vi "Oscillo2graph2024.vi"() -> ()   [LabVIEW 2023]
panel:
  in  "Marker_Size":string
  out "Color Box 5":u32(colorbox)
  out "Color Box 4":u32(colorbox)
  out "Color Box 3":u32(colorbox)
  out "Color Box 2":u32(colorbox)
  out "Color Box":u32(colorbox)
  out "error out":errorcluster
  out "Corner color":u32(colorbox)
  out "Colors traces":string
  out "standard output":string
  out "CLUT":u32[](array[numeric])
  in  "Path":path
  in  "style of points":string
  out "PnG picture":picture
  out "Pixmap vraie couleurs":u32[](array[numeric])
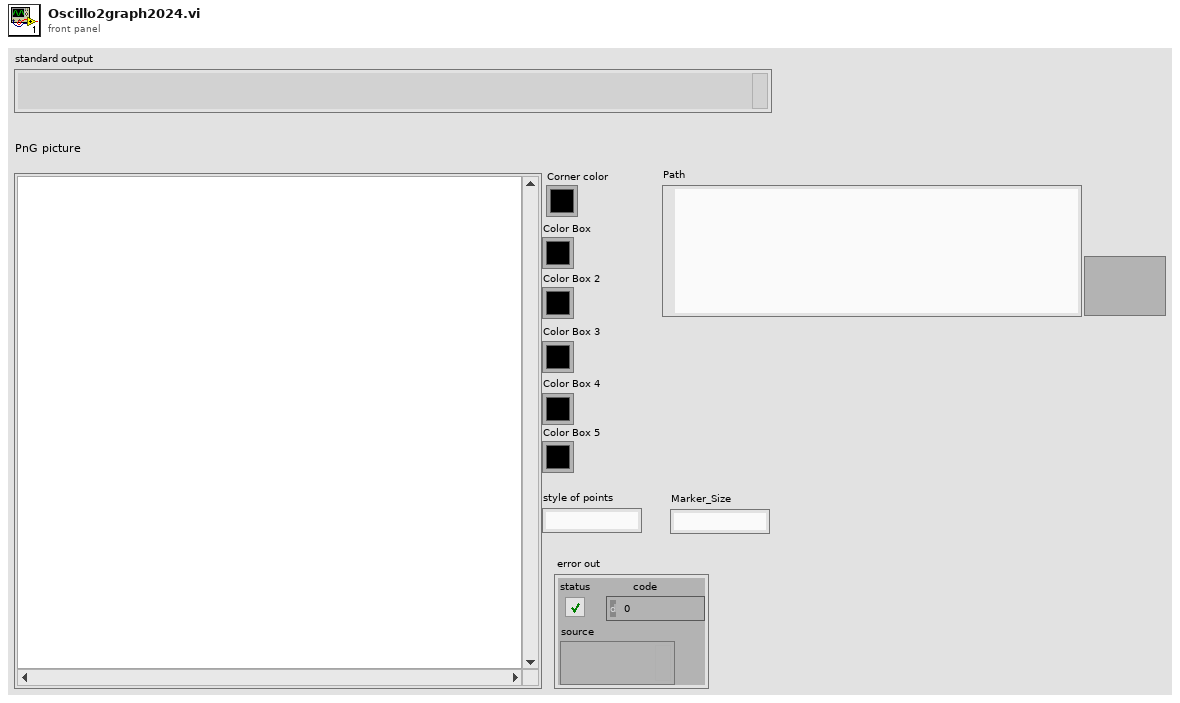
[diagram p1: front panel]
types:
  T1 = cluster{"[0]":u32, "[1]":u32, "[2]":u32, "[3]":u32, "[4]":u32, "[5]":u32, "[6]":u32, "[7]":u32, "[8]":u32}
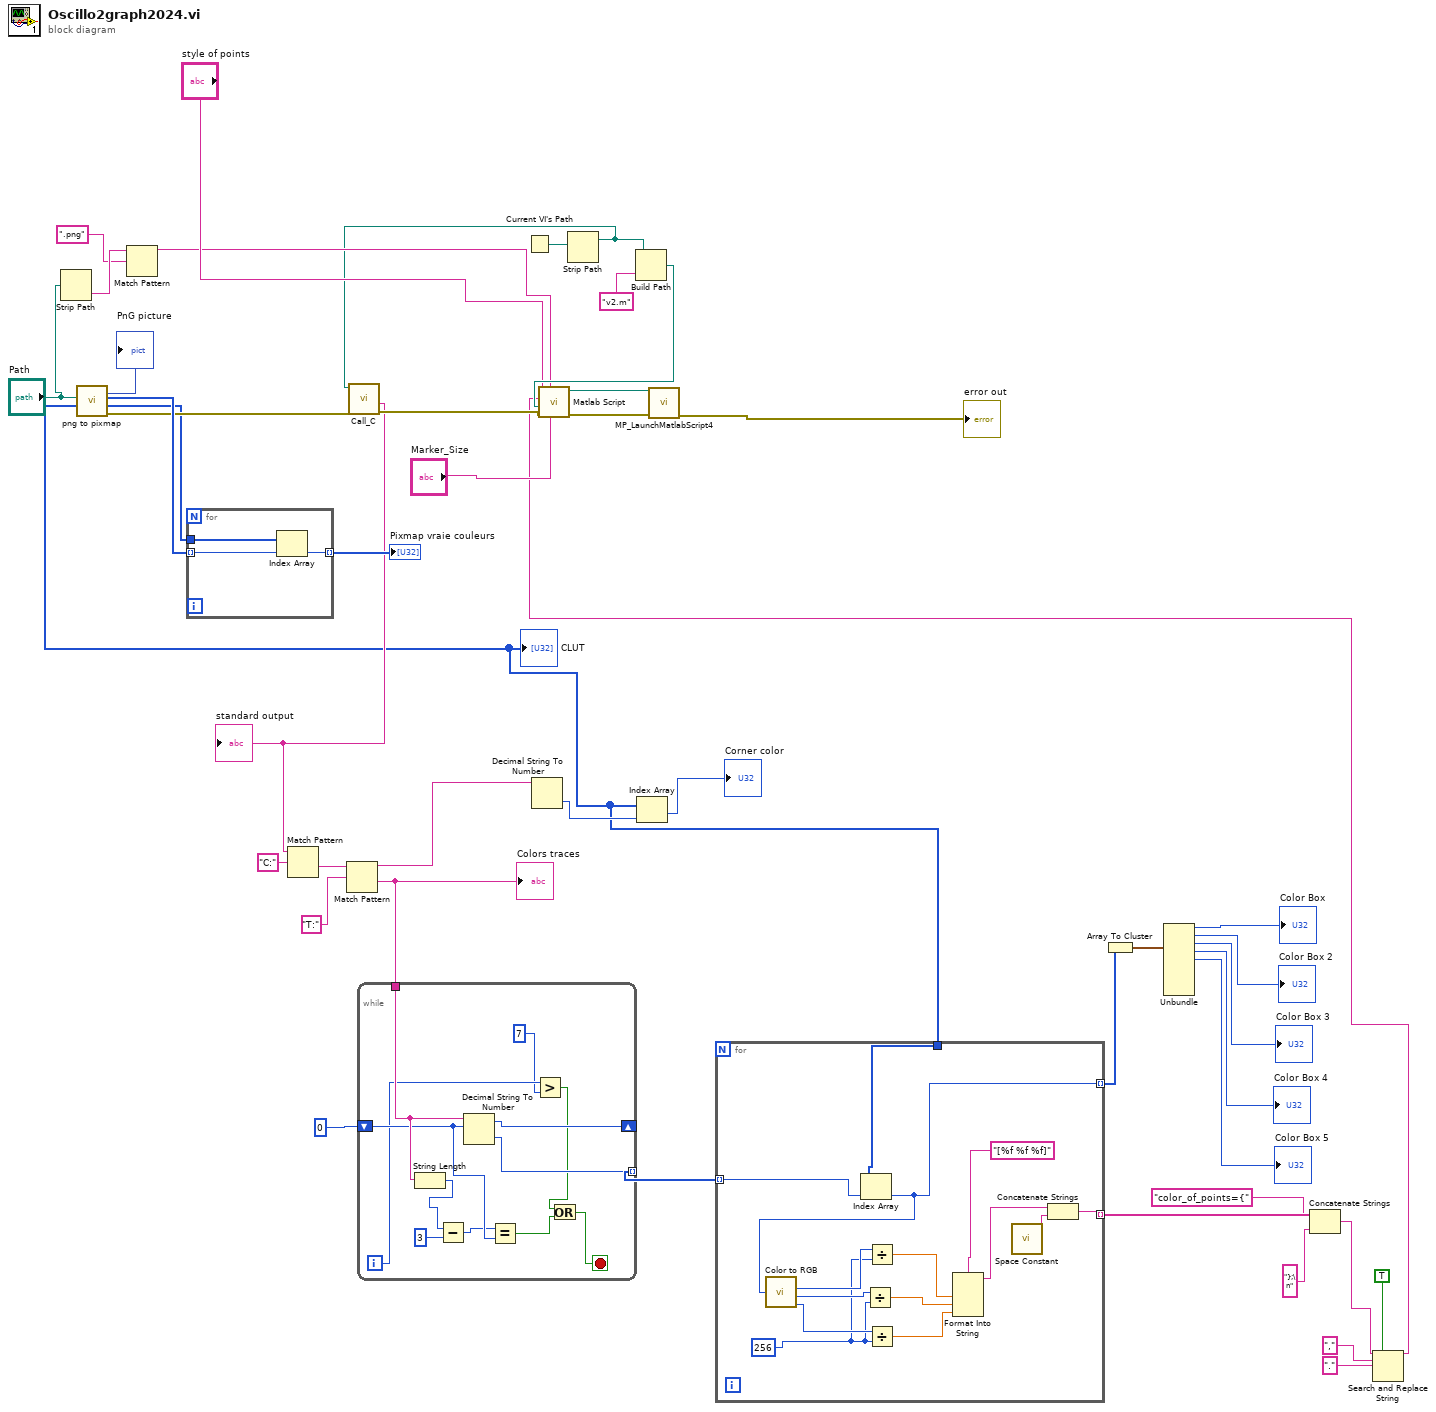
[diagram p0: block diagram]
diagram:
  n1 = Strip Path(path="Path") -> (name=w31:string)  [unwired: 1 out]
  n2 = call "png to pixmap.vi"("Path"="Path") -> ("error out"=w43:errorcluster, "Colors"=w20:u32[], "image"=w44:u8[], "PnG picture"=→"PnG picture":picture)  [unwired: 6 in, 1 out]
  "CLUT" <- w20
  n3 = Match Pattern(string=w31, regular expression=".png") -> (before substring=w29:string)  [unwired: 1 in, 3 out]
  n4 = for {
    tunnel: w44 -> [w46] mode=indexing
    tunnel: [w45] -> w34 mode=indexing
    tunnel: w20 -> [w47]
    n5 = Index Array(array=w47, index=w46) -> (element=w45:u32)
  }
  "Pixmap vraie couleurs" <- w34
  n6 = Current VI's Path() -> (path=w38:path)
  n7 = Strip Path(path=w38) -> (stripped path=w28:path)  [unwired: 1 out]
  n8 = call "Call_C.vi"("error in (no error)"=w43, "working directory"=w28) -> ("error out 2"=w42:errorcluster, "standard output"=w27:string)  [unwired: 7 in, 1 out]
  "standard output" <- w27
  n9 = Match Pattern(string=w27, regular expression="C:") -> (after substring=w25:string)  [unwired: 1 in, 3 out]
  n10 = Match Pattern(string=w25, regular expression="T:") -> (before substring=w23:string, after substring=w15:string)  [unwired: 1 in, 2 out]
  "Colors traces" <- w15
  n11 = while {
    shift-right: [w59] -> _
    shift-left: 0 -> [w56]
    tunnel: w15 -> [w57]
    tunnel: [w58] -> w14 mode=indexing
    i -> [w52]
    stop <- w48 stop-if-true
    n12 = String Length(string=w57) -> (length=w55:i32)
    n13 = Subtract(x=w55, y=3) -> (x-y=w53:i32)
    n14 = Decimal String To Number(string=w57, offset=w56) -> (offset past number=w59:i32, number=w58:i32)  [unwired: 1 in]
    n15 = Equal?(x=w53, y=w56) -> (x = y?=w49:bool)
    n16 = Greater?(x=w52, y=7) -> (0:w50:bool)
    n17 = Or(x=w50, y=w49) -> (x .or. y?=w48:bool)
  }
  n18 = Decimal String To Number(string=w23) -> (number=w22:i32)  [unwired: 2 in, 1 out]
  n19 = Build Path(base path=w28, name or relative path="v2.m") -> (appended path=w36:path)
  n20 = Index Array(array=w20, index=w22) -> (element=→"Corner color":u32)
  n21 = for {
    tunnel: w20 -> [w73]
    tunnel: [w72] -> w19 mode=indexing
    tunnel: w14 -> [w71] mode=indexing
    tunnel: [w62] -> w13 mode=indexing
    w61 = 256
    n22 = Index Array(array=w73, index=w71) -> (element=w62:u32)
    n23 = call <vilib>:"Color to RGB.vi"("Color"=w62) -> ("R"=w64:u8, "G"=w65:u8, "B"=w66:u8)  [unwired: 1 out]
    n24 = Divide(x=w65, y=w61) -> (x/y=w68:dbl)
    n25 = Divide(x=w64, y=w61) -> (x/y=w67:dbl)
    n26 = Divide(x=w66, y=w61) -> (x/y=w69:dbl)
    n27 = Format Into String(format string="[%f %f %f]", w67, w68, w69) -> (resulting string=w63:string)  [unwired: 2 in, 1 out]
    n28 = call <vilib>:"Space Constant.vi"() -> ("String"=w70:string)
    n29 = Concatenate Strings(w63, w70) -> (w72:string)
  }
  n30 = Array To Cluster(array=w13) -> (cluster=w12:T1)
  n31 = Unbundle(w12) -> ("[0]"=→"Color Box":u32, "[1]"=→"Color Box 2":u32, "[2]"=→"Color Box 3":u32, "[3]"=→"Color Box 4":u32, "[4]"=→"Color Box 5":u32)  [unwired: 4 out]
  n32 = Concatenate Strings("color_of_points={" ("string"), w19, "};\n" ("string")) -> (w2:string)
  n33 = Search and Replace String(replace all?=TRUE ("replace all? (F)"), input string=w2, search string=",", replace string="." ("replace string (\"\")")) -> (result string=w1:string)  [unwired: 4 in, 3 out]
  n34 = call "Matlab Script.vi"("Marker_Size"="Marker_Size", "nom source"=w29, "error in"=w42, "path to matlab"=w36, "Color of points"=w1, "style of points"="style of points") -> ("error out"=w41:errorcluster, "path"=w40:path)  [unwired: 4 in]
  n35 = call "MP_LaunchMatlabScript4.vi"("error in (no error)"=w41, "matlab script path"=w40) -> ("error out"=→"error out":errorcluster)  [unwired: 4 in, 5 out]
